vi "updateData.vi"(8 "error in (no error)":errorcluster, 10 "table":T1, 11 "reference in":refnum<class "Items Controller.lvclass">) -> (0 "error out":errorcluster, 3 "reference out":refnum<class "Items Controller.lvclass">)   [LabVIEW 2015, in "Items Controller.lvclass"]
uses:
  Items Controller.lvclass
  APP/checkIN_class/checkIN.lvclass
  APP/checkOUT_class/checkOUT.lvclass
  APP/item_class/item.lvclass
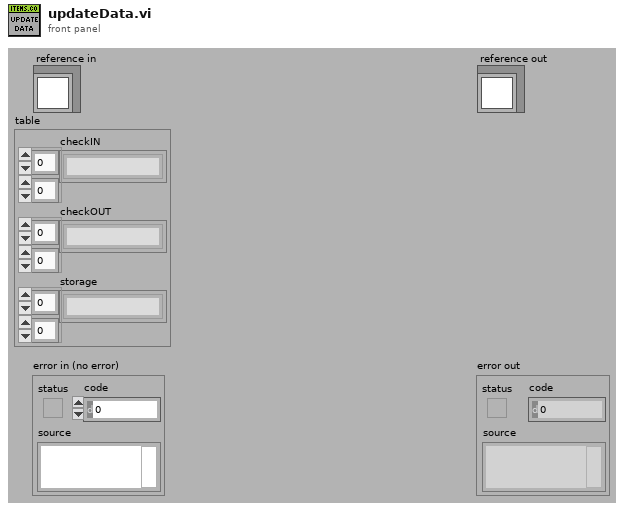
[diagram p1: front panel]
types:
  T1 = cluster{"checkIN":string[][], "checkOUT":string[][], "storage":string[][]}
  T2 = typedef "Items Controller.lvclass/ObjectAttributesRef.ctl" = refnum<data-value>
  T3 = typedef "Items Controller.lvclass/ObjectAttributes.ctl" = cluster{"MyAttribute":dbl, "data":string[][][], "file_controller_ref":refnum<class "File Controller.lvclass">, "checkIN_ref":refnum<class "checkIN.lvclass">, "checkOUT_ref":refnum<class "checkOUT.lvclass">, "item_ref":refnum<class "item.lvclass">}
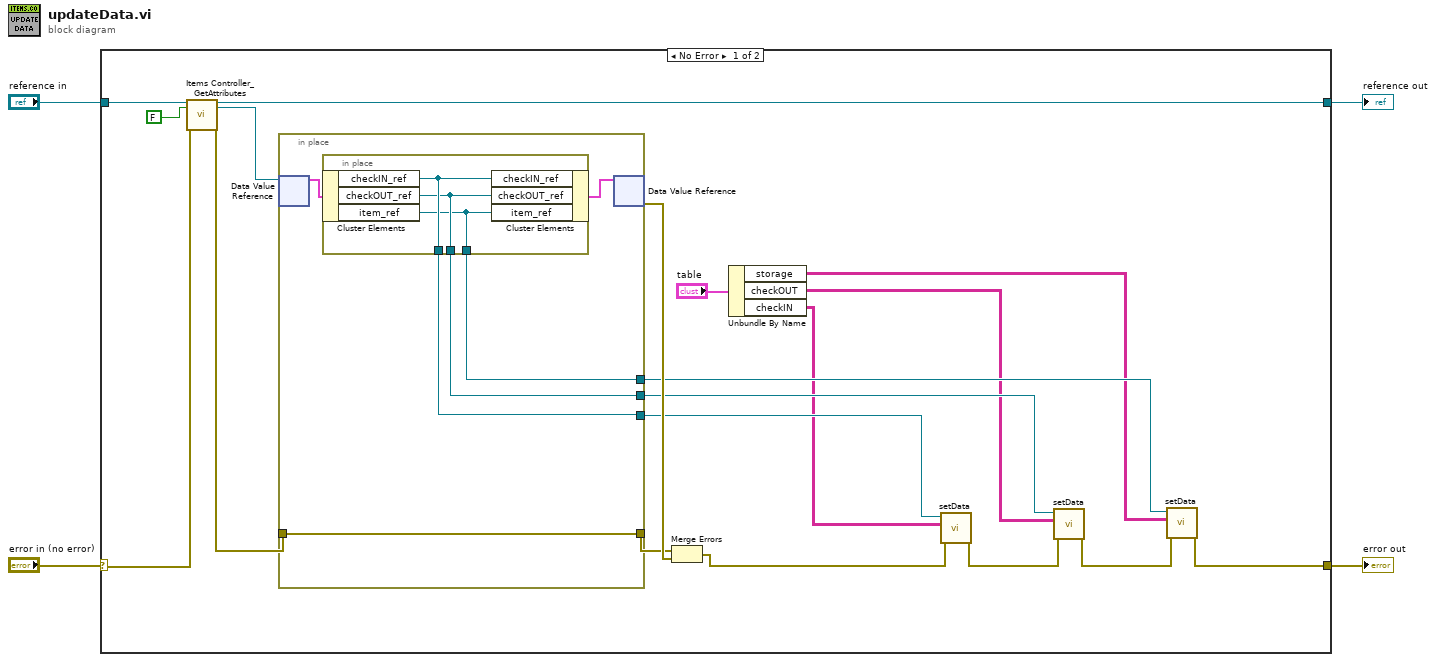
[diagram p0: block diagram]
diagram:
  n1 = case shown="No Error" "error in (no error)" {
    selector: "error in (no error)" -> [w19 w34]
    tunnel: [w9 w34] -> w3
    tunnel: [w17 w33] -> w1
    tunnel: "reference in" -> [w21 w33]
    frame No Error {
      n2 = call "Items Controller_GetAttributes.vi"("reference in"=w21, "return data? (T)"=FALSE, "error in (no error)"=w19) -> ("reference out"=w17:refnum<class "Items Controller.lvclass">, "attributes ref"=w16:T2, "error out"=w18:errorcluster)  [unwired: 13 in, 1 out]
      n3 = in-place {
        in-place-border: w18 -> [w27]
        in-place-border: [w27] -> w22
        in-place-border: [w26] -> w13
        in-place-border: [w25] -> w12
        in-place-border: [w24] -> w11
        n4 = in-place-dvr #1(w16) -> (w28:T3)  [unwired: 1 out]
        n5 = in-place {
          in-place-border: [w32] -> w26
          in-place-border: [w31] -> w25
          in-place-border: [w30] -> w24
          n6 = in-place-cluster #2(w28) -> ("checkIN_ref"=w32:refnum<class "checkIN.lvclass">, "checkOUT_ref"=w31:refnum<class "checkOUT.lvclass">, "item_ref"=w30:refnum<class "item.lvclass">)
          n7 = in-place-cluster #2("checkIN_ref"=w32, "checkOUT_ref"=w31, "item_ref"=w30) -> (w29:T3)
        }
        n8 = in-place-dvr #1(w29) -> (w23:errorcluster)  [unwired: 1 out]
      }
      n9 = Merge Errors(w22, w23) -> (w15:errorcluster)
      n10 = Unbundle By Name("table") -> ("storage"=w5:string[][], "checkOUT"=w6:string[][], "checkIN"=w7:string[][])
      n11 = call "setData.vi"("error in (no error)"=w15, "data"=w7, "reference in"=w13) -> ("error out"=w14:errorcluster)  [unwired: 7 in, 1 out]
      n12 = call "setData.vi"("error in (no error)"=w14, "data"=w6, "reference in"=w12) -> ("error out"=w10:errorcluster)  [unwired: 7 in, 1 out]
      n13 = call "setData.vi"("error in (no error)"=w10, "data"=w5, "reference in"=w11) -> ("error out"=w9:errorcluster)  [unwired: 7 in, 1 out]
    }
    frame Error {
    }
  }
  "error out" <- w3
  "reference out" <- w1
